vi "iWorx Snapshot.vi"(8 "Error In":errorcluster, 11 "WaveformChart in":refnum<vi>) -> (0 "Error Out":errorcluster)   [LabVIEW 2014]
doc: "This VI is designed to take a screenshot of a waveform chart (specified by reference), and prompt to user to save it on disc."
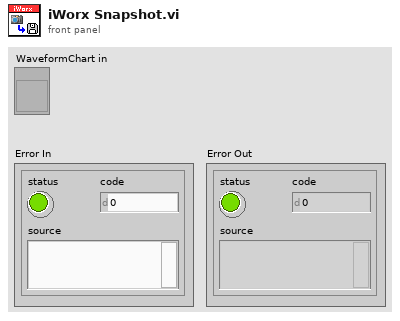
[diagram p1: front panel]
types:
  T1 = enum16{"open", "replace", "create", "open or create", "replace or create", "replace or create with confirmation"}
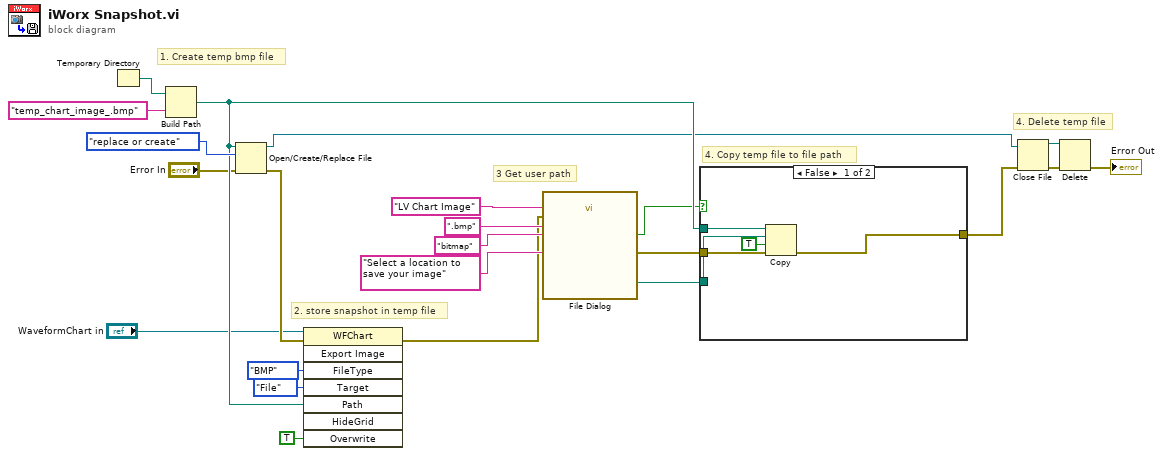
[diagram p0: block diagram]
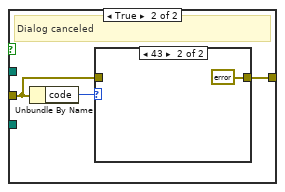
[diagram p2: hidden frame]
diagram:
  # "3 Get user path"
  # "4. Delete temp file"
  # "4. Copy temp file to file path"
  # "2. store snapshot in temp file"
  # "1. Create temp bmp file"
  n1 = Temporary Directory() -> (w6:path)
  n2 = Build Path(base path=w6, name or relative path="temp_chart_image_.bmp") -> (appended path=w13:path)
  n3 = Open/Create/Replace File(file path (use dialog)=w13, error in="Error In", operation (0:open)=T1."replace or create") -> (refnum out=w10:refnum<file>, error out=w19:errorcluster)  [unwired: 3 in, 1 out]
  n4 = invoke on="Invoke Node" class="WFChart" method="Export Image"(reference="WaveformChart in", error in=w19, "FileType"=enum32{"BMP", "EPS", "EMF", "PICT"}."BMP" ("File Type"), "Target"=enum32{"File", "Clipboard"}."File", "Path"=w13, "Overwrite"=TRUE ("Always Overwrite")) -> (error out=w14:errorcluster)  [unwired: 2 in, 7 out]
  n5 = call "File Dialog"("prompt"="Select a location to save your image", "default name"="LV Chart Image", "error in"=w14, "pattern (all files)"=".bmp", "pattern label"="bitmap") -> ("selected path"=w12:path, "cancelled"=w4:bool, "error out"=w11:errorcluster)  [unwired: 7 in, 1 out]
  n6 = case shown="False" w4 {
    tunnel: w13 -> [w28 _]
    tunnel: w12 -> [w27 _]
    tunnel: w11 -> [w26 w30]
    tunnel: [w25 w29] -> w9
    frame False {
      n7 = Copy(8:w26, 9:TRUE ("overwrite (F)"), 10:w27, 11:w28) -> (0:w25:errorcluster)  [unwired: 1 in, 2 out]
    }
    frame True {
      # "Dialog canceled"
      n8 = Unbundle By Name(w30) -> ("code"=w31:i32)
      n9 = case shown="43" w31 {
        tunnel: w30 -> [w32 _]
        tunnel: [w32 errorcluster {"status"=FALSE, "code"=0, "source"=""} ("error out")] -> w29
        frame 0, Default {
        }
        frame 43 {
        }
      }
    }
  }
  n10 = Close File(refnum=w10, error in=w9) -> (path=w8:path, error out=w7:errorcluster)
  n11 = Delete(path (use dialog)=w8, error in=w7) -> (error out=→"Error Out":errorcluster)  [unwired: 3 in, 2 out]
